vi "ROTATE KICKER.vi"(8 "error in (no error)":errorcluster, 9 "RefName COUNT":string="KICKERCOUNT", 10 "RefName KICKER":string="KICKER") -> (0 "error out":errorcluster)   [LabVIEW 2020]
panel:
  in  "Use HALL counter?":bool
  out "msec per rev":dbl
  out "final rpm":dbl
  in  "motor speed (rpm)":dbl=24.0 format="%#_13g"
  in  "kicker speed":dbl=1.0 min=-1.0 max=1.0 step=0.1 format="%.3g"
  out "count":i32
  out "target count":dbl
  in  "KICKER REVOLUTIONS":dbl=2.0 format="%#_13g"
  out "start count":i32
  out "final gearing":dbl
  in  "TEETH - shaft":dbl=17.0
  in  "TEETH - pinion":dbl=17.0
  in  "gear ratio":dbl=174.9
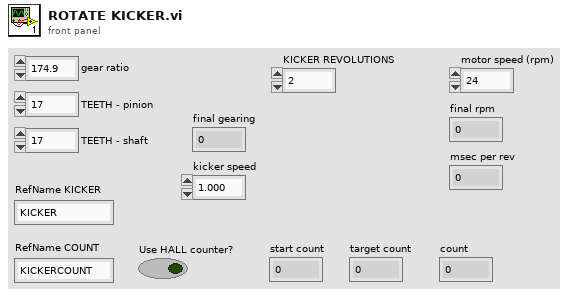
[diagram p1: front panel]
types:
  T1 = typedef "WPI_SwitchDevRef.ctl" = cluster{"DevStatus":errorcluster, "DIO Channel":T2, "CntIndex":T3, "Normally Closed":bool}
  T2 = typedef "FPGA_DIOChannel.ctl" = enum8{"DIO 0", "DIO 1", "DIO 2", "DIO 3", "DIO 4", "DIO 5", "DIO 6", "DIO 7", "DIO 8", "DIO 9", "DIO MXP 0", "DIO MXP 1", "DIO MXP 2", "DIO MXP 3", "DIO MXP 4", "DIO MXP 5", "DIO MXP 6", "DIO MXP 7", "DIO MXP 8", "DIO MXP 9", "DIO MXP 10", "DIO MXP 11", "DIO MXP 12", "DIO MXP 13", "DIO MXP 14", "DIO MXP 15", "SPI Port CS1", "SPI Port CS2", "SPI Port CS3", "SPI Port MISO", "SPI Port MOSI", "Invalid"}
  T3 = typedef "FPGA_CounterCtrSystemIndex.ctl" = enum8{"Ctr 0", "Ctr 1", "Ctr 2", "Ctr 3", "Ctr 4", "Ctr 5", "Ctr 6", "Ctr 7", "Invalid"}
  T4 = typedef "WPI_MotorControlDeviceRef.ctl" = cluster{"DeviceStatus":errorcluster, "Type":T5, "PWM":cluster{"PWM Channel":T6, "DeadBand":T7}, "CAN":cluster{"Device Number":u8, "SetOutput VI Ref":variant, "GetOutput VI Ref":variant, "Enable VI Ref":variant, "Disable VI Ref":variant, "Data":variant}, "Invert":bool, "DIO PWM":cluster{"PWM \"Enable\" Channel":T6, "DIOChannel":T2, "PWM Rate":dbl}}
  T5 = typedef "WPI_MotorControlType.ctl" = enum16{"PWM", "CAN", "DIO PWM"}
  T6 = typedef "FPGA_DIOPWMChannel.ctl" = enum8{"PWM 0", "PWM 1", "PWM 2", "PWM 3", "PWM 4", "PWM 5", "PWM 6", "PWM 7", "PWM 8", "PWM 9", "PWM MXP 0", "PWM MXP 1", "PWM MXP 2", "PWM MXP 3", "PWM MXP 4", "PWM MXP 5", "PWM MXP 6", "PWM MXP 7", "PWM MXP 8", "PWM MXP 9", "Invalid"}
  T7 = typedef "WPI_PWMDeadband.ctl" = cluster{"Name":string, "maxPositivePwm":i32, "minPositivePwm":i32, "centerPwm":i32, "maxNegativePwm":i32, "minNegativePwm":i32, "angularRange":u16}
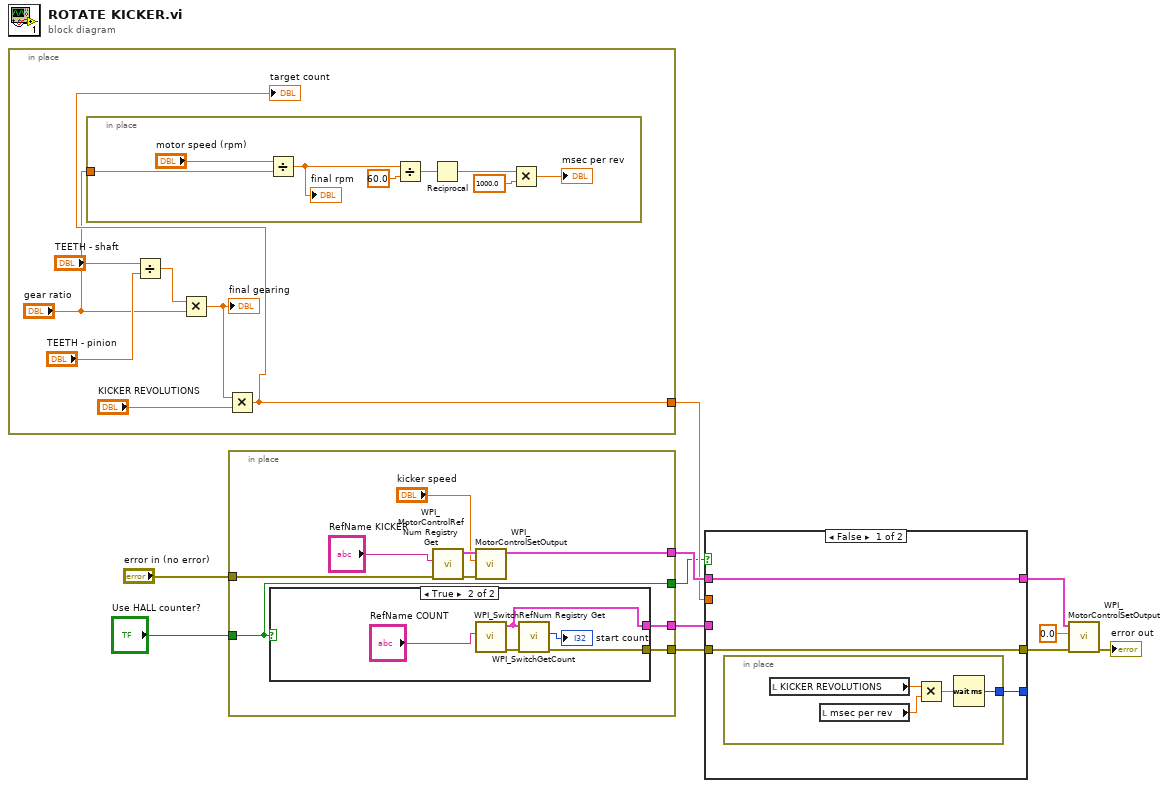
[diagram p0: block diagram]
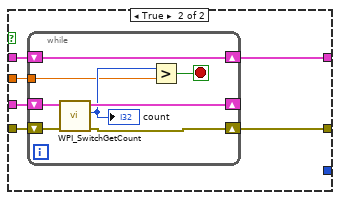
[diagram p2: hidden frame]
diagram:
  n1 = in-place {
    in-place-border: [w13] -> w5
    n2 = in-place {
      in-place-border: "gear ratio" -> [w25]
      n3 = Divide(x="motor speed (rpm)", y=w25) -> (x/y=w24:dbl)
      "final rpm" <- w24
      n4 = Divide(x=w24, y=60.0) -> (x/y=w22:dbl)
      n5 = Reciprocal(x=w22) -> (1/x=w21:dbl)
      n6 = Multiply(x=w21, y=1000.0) -> (x*y=→"msec per rev":dbl)
    }
    n7 = Divide(x="TEETH - shaft", y="TEETH - pinion") -> (x/y=w16:dbl)
    n8 = Multiply(x=w16, y="gear ratio") -> (x*y=w15:dbl)
    "final gearing" <- w15
    n9 = Multiply(x=w15, y="KICKER REVOLUTIONS") -> (x*y=w13:dbl)
    "target count" <- w13
  }
  n10 = in-place {
    in-place-border: [w31] -> w11
    in-place-border: [w30] -> w9
    in-place-border: [w29] -> w8
    in-place-border: "error in (no error)" -> [w28]
    in-place-border: [w27] -> w2
    in-place-border: "Use HALL counter?" -> [w27]
    n11 = case shown="True" w27 {
      tunnel: [_ w37] -> w30
      tunnel: [_ w36] -> w29
      frame False {
      }
      frame True {
        n12 = call <vilib>:"WPI_SwitchRefNum Registry Get.vi"("refnum name"="RefName COUNT") -> ("error out"=w39:errorcluster, "SwitchDevRef"=w37:T1)  [unwired: 9 in]
        n13 = call <vilib>:"WPI_SwitchGetCount.vi"("error in (no error)"=w39, "SwitchDevRef"=w37) -> ("error out"=w36:errorcluster, "Switch Pressed Count"=→"start count":i32)  [unwired: 7 in, 1 out]
      }
    }
    n14 = call <vilib>:"WPI_MotorControlRefNum Registry Get.vi"("error in (no error)"=w28, "refnum name"="RefName KICKER") -> ("error out"=w34:errorcluster, "MotorControlDevRef"=w33:T4)  [unwired: 8 in]
    n15 = call <vilib>:"WPI_MotorControlSetOutput.vi"("error in (no error)"=w34, "Output"="kicker speed", "MotorControlDevRef"=w33) -> ("MotorControlDevRef"=w31:T4)  [unwired: 6 in, 2 out]
  }
  n16 = case shown="False" w2 {
    tunnel: w11 -> [w41 w53]
    tunnel: [w41 w52] -> w10
    tunnel: w9 -> [_ w51]
    tunnel: w8 -> [w42 w50]
    tunnel: [w42 w49] -> w7
    tunnel: w5 -> [_ w48]
    tunnel: [w43 _] -> _
    frame False {
      n17 = in-place {
        in-place-border: [w47] -> w43
        n18 = local read "KICKER REVOLUTIONS"() -> (w45:dbl)
        n19 = local read "msec per rev"() -> (w44:dbl)
        n20 = Multiply(x=w45, y=w44) -> (x*y=w46:dbl)
        n21 = Wait (ms)(milliseconds to wait=w46) -> (millisecond timer value=w47:u32)
      }
    }
    frame True {
      n22 = while {
        shift-right: [w61] -> w52
        shift-left: w53 -> [w61]
        shift-right: [w57] -> w49
        shift-left: w50 -> [w59]
        shift-right: [w58] -> _
        shift-left: w51 -> [w60]
        tunnel: w48 -> [w54]
        stop <- w55 stop-if-true
        n23 = call <vilib>:"WPI_SwitchGetCount.vi"("error in (no error)"=w59, "SwitchDevRef"=w60) -> ("error out"=w57:errorcluster, "Switch Pressed Count"=w56:i32, "SwitchDevRef"=w58:T1)  [unwired: 7 in]
        "count" <- w56
        n24 = Greater?(x=w56, y=w54) -> (0:w55:bool)
      }
    }
  }
  n25 = call <vilib>:"WPI_MotorControlSetOutput.vi"("error in (no error)"=w7, "Output"=0.0, "MotorControlDevRef"=w10) -> ("error out"=→"error out":errorcluster)  [unwired: 6 in, 2 out]
